vi "Home Location.vi"(7 "Method":enum16{"Get", "Set"}(ring), 8 "error in (no error)":errorcluster, 9 "Longitude In":dbl, 10 "Latitude In":dbl, 11 "config refnum":T1) -> (0 "error out":errorcluster, 1 "Longitude Out":dbl, 2 "Latitude Out":dbl, 3 "refnum out":T1)   [LabVIEW 2014]
uses:
  <vilib>/Utility/config.llb/Config Data RefNum.ctl
  <vilib>/Utility/config.llb/Read Key (Double).vi
  <vilib>/Utility/config.llb/Write Key (Double).vi
  <vilib>/Utility/config.llb/NI_LVConfig.lvlib
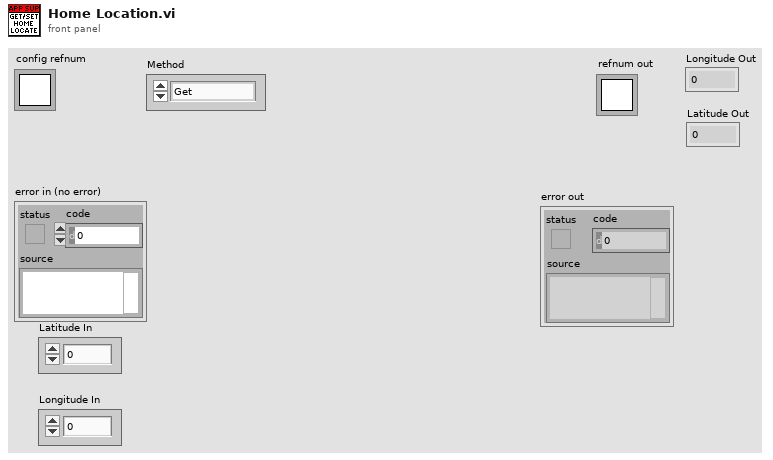
[diagram p1: front panel]
types:
  T1 = typedef "NI_LVConfig.lvlib/Config Data RefNum.ctl" = refnum<k1>
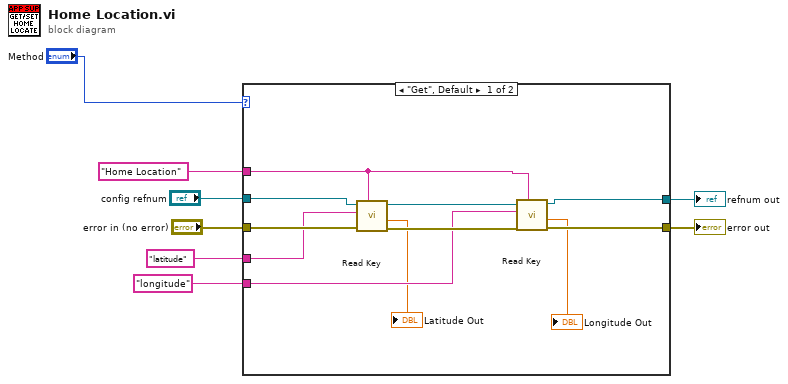
[diagram p0: block diagram]
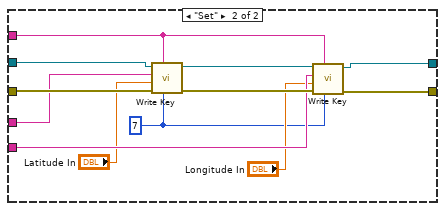
[diagram p2: hidden frame]
diagram:
  n1 = case shown="\"Get\", Default" "Method" {
    tunnel: "error in (no error)" -> [w18 w30]
    tunnel: [w17 w21] -> w6
    tunnel: "Home Location" ("section") -> [w16 w27]
    tunnel: "config refnum" -> [w15 w31]
    tunnel: "latitude" ("key") -> [w13 w26]
    tunnel: "longitude" ("key") -> [w12 w25]
    tunnel: [w9 w22] -> w1
    frame "Get", Default {
      n2 = call-poly <vilib>:"Read Key.vi"("section"=w16, "error in (no error)"=w18, "key"=w13, "refnum"=w15) -> ("error out"=w19:errorcluster, "value"=→"Latitude Out":dbl, "refnum out"=w14:T1)  [unwired: 4 in, 1 out]
      n3 = call-poly <vilib>:"Read Key.vi"("section"=w16, "error in (no error)"=w19, "key"=w12, "refnum"=w14) -> ("error out"=w17:errorcluster, "value"=→"Longitude Out":dbl, "refnum out"=w9:T1)  [unwired: 4 in, 1 out]
    }
    frame "Set" {
      w20 = i16 7 ("precision (6)")
      n4 = call-poly <vilib>:"Write Key.vi"("precision (6)"=w20, "section"=w27, "error in (no error)"=w30, "value"="Latitude In", "key"=w26, "refnum"=w31) -> ("error out"=w29:errorcluster, "refnum out"=w28:T1)  [unwired: 3 in, 1 out]
      n5 = call-poly <vilib>:"Write Key.vi"("precision (6)"=w20, "section"=w27, "error in (no error)"=w29, "value"="Longitude In", "key"=w25, "refnum"=w28) -> ("error out"=w21:errorcluster, "refnum out"=w22:T1)  [unwired: 3 in, 1 out]
    }
  }
  "error out" <- w6
  "refnum out" <- w1
